vi "Rn.vi"(2 "Collector Area (Ac)":dbl, 3 "Nozzle Area (An)":dbl) -> (0 "Equivalent Collector Radius (Rc)":dbl, 1 "Equivalent Nozzle Radius (Rn)":dbl)   [LabVIEW 2017]
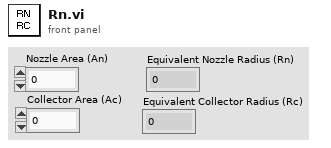
[diagram p1: front panel]
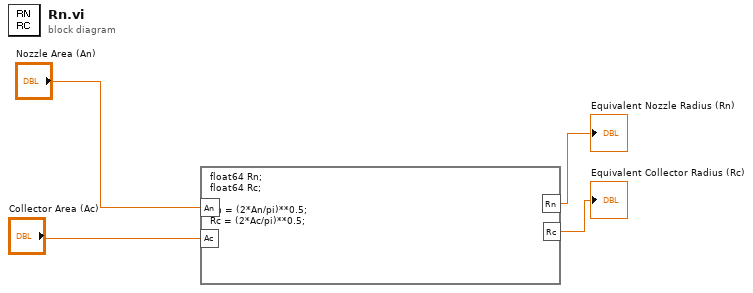
[diagram p0: block diagram]
diagram:
  n1 = formula code="float64 Rn;\nfloat64 Rc;\n\nRn = (2*An/pi)**0.5;\nRc = (2*Ac/pi)**0.5;"("An"="Nozzle Area (An)", "Ac"="Collector Area (Ac)") -> ("Rn"=→"Equivalent Nozzle Radius (Rn)":dbl, "Rc"=→"Equivalent Collector Radius (Rc)":dbl)
